vi "EnterOrExitRandom.vi"(8 "In (T) / Out (F)":bool=TRUE, 9 "Occup array":refnum<vi>[](array[refnum]), 10 "Sense array":refnum<vi>[](array[refnum]), 11 "Occupancy in":T2) -> (3 "Occupancy out":T1)   [LabVIEW 2023]
uses:
  <vilib>/numeric/Random Number (Range) U64.vi
  <vilib>/numeric/sub_Random U32.vi
  <userlib>/_OpenG.lib/array/array.llb/Search 1D Array (Boolean)__ogtk.vi
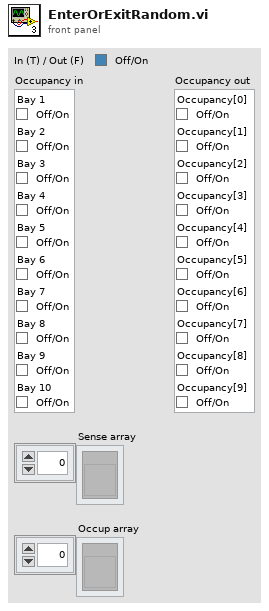
[diagram p1: front panel]
types:
  T1 = cluster{"Occupancy[0]":bool, "Occupancy[1]":bool, "Occupancy[2]":bool, "Occupancy[3]":bool, "Occupancy[4]":bool, "Occupancy[5]":bool, "Occupancy[6]":bool, "Occupancy[7]":bool, "Occupancy[8]":bool, "Occupancy[9]":bool}
  T2 = cluster{"Bay 1":bool, "Bay 2":bool, "Bay 3":bool, "Bay 4":bool, "Bay 5":bool, "Bay 6":bool, "Bay 7":bool, "Bay 8":bool, "Bay 9":bool, "Bay 10":bool}
  T3 = cluster{"Occupancy in[0]":bool, "Occupancy in[1]":bool, "Occupancy in[2]":bool, "Occupancy in[3]":bool, "Occupancy in[4]":bool, "Occupancy in[5]":bool, "Occupancy in[6]":bool, "Occupancy in[7]":bool, "Occupancy in[8]":bool, "Occupancy in[9]":bool}
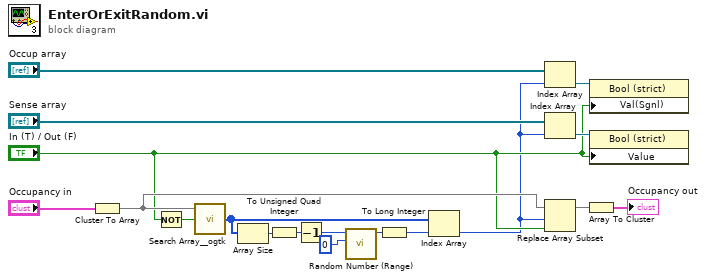
[diagram p0: block diagram]
diagram:
  n1 = Cluster To Array(cluster="Occupancy in") -> (array=w17:bool[])
  n2 = Not(x="In (T) / Out (F)") -> (.not. x?=w5:bool)
  n3 = call-poly <userlib>:"Search Array__ogtk.vi"("Array"=w17, "Element Data"=w5) -> ("Indices of Elements"=w3:i32[])  [unwired: 7 in]
  n4 = Array Size(array=w3) -> (size(s)=w16:i32)
  n5 = To Unsigned Quad Integer(1:w16) -> (0:w15:u64)
  n6 = Decrement(x=w15) -> (x-1=w4:u64)
  n7 = call-poly <vilib>:"Random Number (Range).vi"("lower bound (0)"=u64 0, "upper bound (100)"=w4) -> ("number"=w13:u64)  [unwired: 9 in]
  n8 = To Long Integer(number=w13) -> (32bit integer=w2:i32)
  n9 = Index Array(array=w3, index=w2) -> (element=w1:i32)
  n10 = Index Array(array="Occup array", index=w1) -> (element=w9:refnum<vi>)
  n11 = Index Array(array="Sense array", index=w1) -> (element=w7:refnum<vi>)
  n12 = Replace Array Subset(array=w17, new element="In (T) / Out (F)", index=w1) -> (w11:bool[])
  n13 = Array To Cluster(array=w11) -> (cluster=→"Occupancy out":T3)
  n14 = property class="Bool (strict)"(reference=w9, "Val(Sgnl)"="In (T) / Out (F)") -> ()  [unwired: 1 in, 2 out]
  n15 = property class="Bool (strict)"(reference=w7, "Value"="In (T) / Out (F)") -> ()  [unwired: 1 in, 2 out]
